vi "Create Lines for Table.vi"(0 "versions":T1, 1 "Devices WhoAmI List":u16[](array[numeric])=[0, 1024, 1040, 1056, 1072, 1088, 1104, 1121, 1136, 1152, 1168, 1216], 2 "Devices Name List":string[](array[string])=["Not defined", "Poke", "Multi Pwm Generator", "Wear", "12 Volts Drive", "LED Controller", "Synchronizer", "Simple Analog Generator", "Archimedes", "Clock Synchronizer", "Camera Controller", "Behavior"], 7 "connection type":string) -> (8 "line":string[](array[string]))   [LabVIEW 2010]
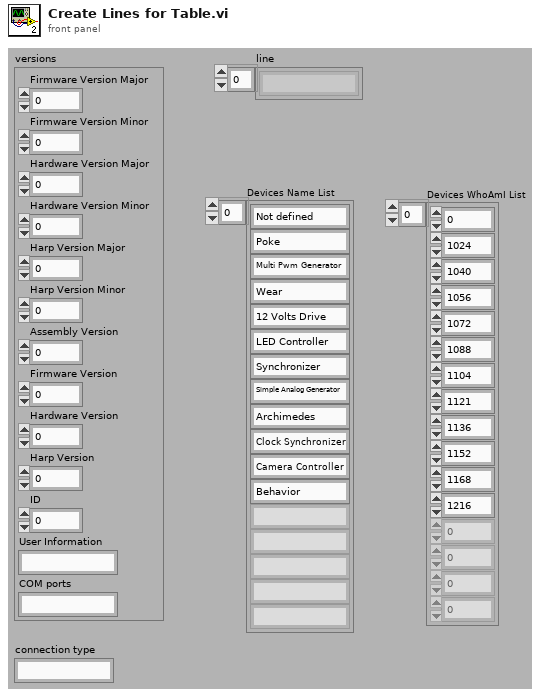
[diagram p1: front panel]
types:
  T1 = cluster{"Firmware Version Major":u8, "Firmware Version Minor":u8, "Hardware Version Major":u8, "Hardware Version Minor":u8, "Harp Version Major":u8, "Harp Version Minor":u8, "Assembly Version":u8, "Firmware Version":dbl, "Hardware Version":dbl, "Harp Version":dbl, "ID":u16, "User Information":string, "COM ports":string}
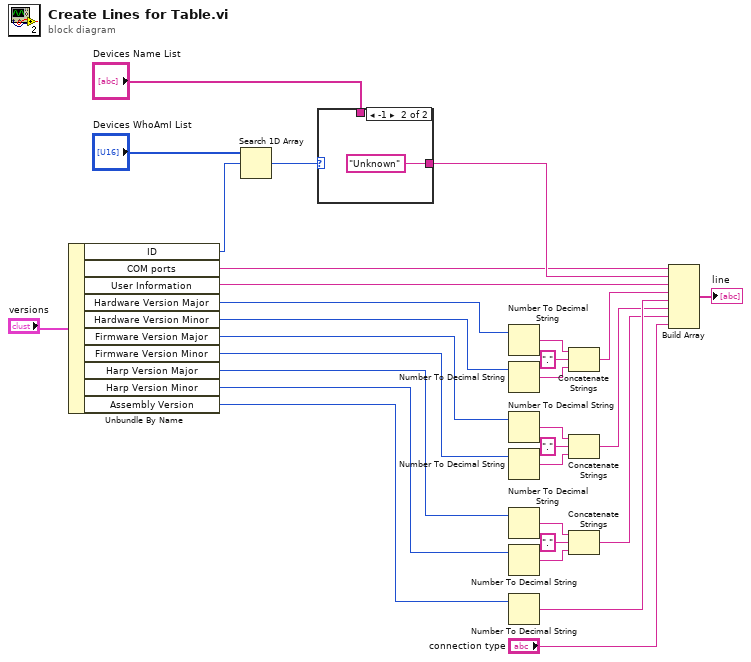
[diagram p0: block diagram]
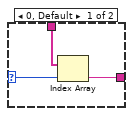
[diagram p2: hidden frame]
diagram:
  n1 = Unbundle By Name("versions") -> ("ID"=w9:u16, "COM ports"=w10:string, "User Information"=w12:string, "Hardware Version Major"=w13:u8, "Hardware Version Minor"=w14:u8, "Firmware Version Major"=w21:u8, "Firmware Version Minor"=w22:u8, "Harp Version Major"=w26:u8, "Harp Version Minor"=w27:u8, "Assembly Version"=w28:u8)
  n2 = Search 1D Array(1D array="Devices WhoAmI List", element=w9) -> (index of element=w6:i32)  [unwired: 1 in]
  n3 = case shown="-1" w6 {
    selector: w6 -> [w31 _]
    tunnel: [w33 "Unknown" ("message")] -> w11
    tunnel: "Devices Name List" -> [w32 _]
    frame 0, Default {
      n4 = Index Array(array=w32, index=w31) -> (element=w33:string)
    }
    frame -1 {
    }
  }
  n5 = Number To Decimal String(number=w13) -> (decimal integer string=w15:string)  [unwired: 1 in]
  n6 = Number To Decimal String(number=w14) -> (decimal integer string=w16:string)  [unwired: 1 in]
  n7 = Number To Decimal String(number=w21) -> (decimal integer string=w20:string)  [unwired: 1 in]
  n8 = Number To Decimal String(number=w22) -> (decimal integer string=w19:string)  [unwired: 1 in]
  n9 = Number To Decimal String(number=w26) -> (decimal integer string=w23:string)  [unwired: 1 in]
  n10 = Number To Decimal String(number=w27) -> (decimal integer string=w24:string)  [unwired: 1 in]
  n11 = Number To Decimal String(number=w28) -> (decimal integer string=w4:string)  [unwired: 1 in]
  n12 = Concatenate Strings(w15, "." ("string"), w16) -> (w5:string)
  n13 = Concatenate Strings(w20, "." ("string"), w19) -> (w3:string)
  n14 = Concatenate Strings(w23, "." ("string"), w24) -> (w2:string)
  n15 = Build Array(w10, w11, w12, w5, w4, w3, w2, "connection type") -> (→"line":string[])
